vi "MultiSetAndClear.vi"(9 "Bits_To_Clear":u8[](array[numeric])=[3], 10 "Bits_To_Set":u8[](array[numeric])=[1, 2], 11 "Data_in":u16) -> (3 "Data_Out":u16)   [LabVIEW 2017, in "Bit Manipulation.lvlib"]
uses:
  Bit Manipulation.lvlib
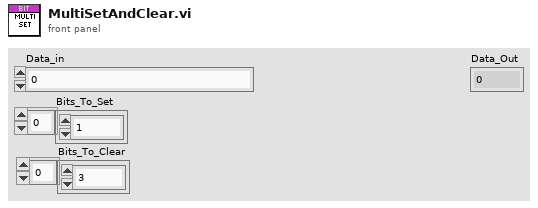
[diagram p1: front panel]
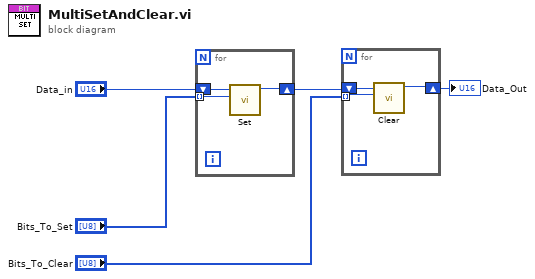
[diagram p0: block diagram]
diagram:
  n1 = for {
    shift-right: [w7] -> w4
    shift-left: "Data_in" -> [w8]
    tunnel: "Bits_To_Set" -> [w6] mode=indexing
    n2 = call "Set.vi"("Bit to set"=w6, "Data_In"=w8) -> ("Data_Out"=w7:u16)  [unwired: 9 in]
  }
  n3 = for {
    shift-right: [w10] -> w1
    shift-left: w4 -> [w11]
    tunnel: "Bits_To_Clear" -> [w9] mode=indexing
    n4 = call "Clear.vi"("Bit to clear"=w9, "Data_In"=w11) -> ("Data_Out"=w10:u16)  [unwired: 9 in]
  }
  "Data_Out" <- w1
